vi "Periodic Tasks.vi"() -> ()   [LabVIEW 2011]
doc: "This VI runs in parallel to other tasks. It can contain as many user-defined periodic loops as you need. These can carry out PID or other sorts of timed response."
uses:
  <vilib>/Rock Robotics/SystemInterfaces/Utilities/FPGA_UtilitiesLED State.ctl
  <vilib>/Rock Robotics/SystemInterfaces/Utilities/FPGA_UtilitiesLED Source.ctl
  Robot Global Data.vi
  <vilib>/Rock Robotics/WPI/Relay/WPI_RelayValue.ctl
panel:
  in  "Speed of Harvester":dbl
  in  "Speed of Conveyor":dbl
  out "Rate 3":dbl
  out "error out 4":errorcluster
  out "Direction 3":bool
  out "Distance 3":dbl
  out "Distance 2":dbl
  out "Direction 2":bool
  out "error out 3":errorcluster
  out "Rate 2":dbl
  out "Rate":dbl
  out "error out 2":errorcluster
  out "I2C":bool
  out "Angular Rate":dbl
  out "Angle":dbl
  out "Direction":bool
  out "Distance":dbl
  # "Target Tracking"
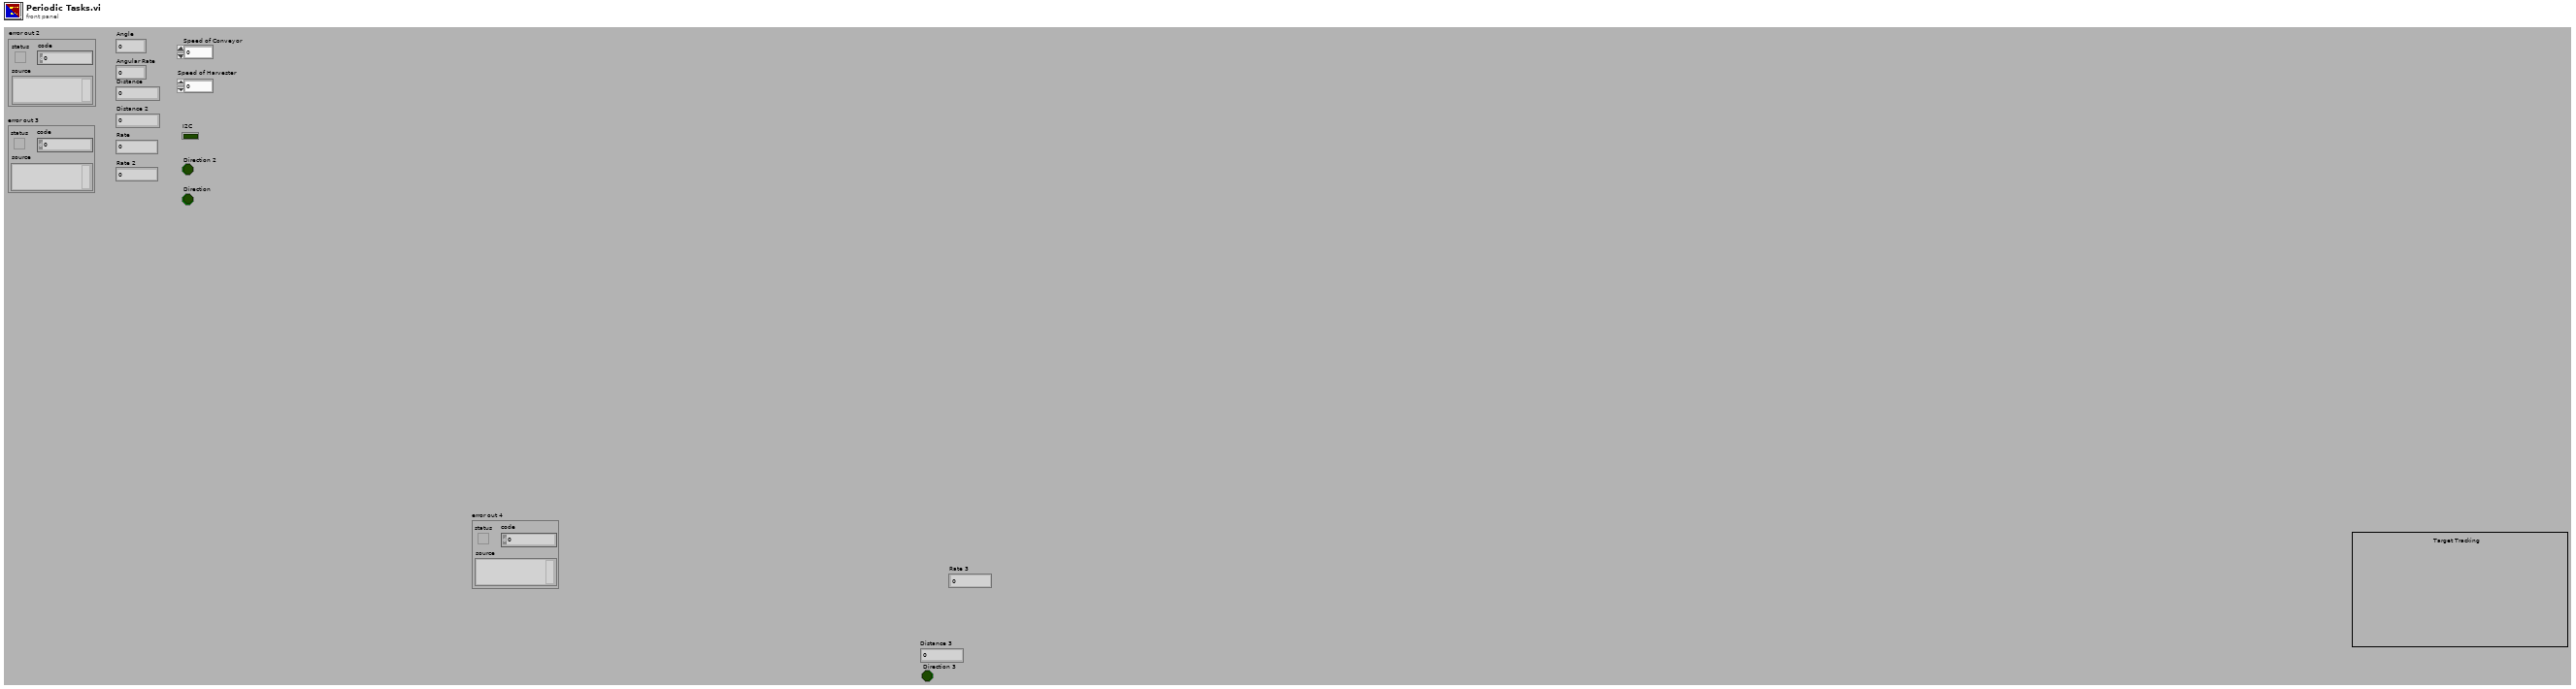
[diagram p1: front panel]
types:
  T1 = typedef "WPI_RelayValue.ctl" = enum16{"Off", "On", "Forward", "Reverse"}
  T2 = typedef "WPI_AnalogChannelDevRef.ctl" = cluster{"DevStatus":errorcluster, "Analog Module":T3, "Analog Channel":T4}
  T3 = typedef "FPGA_TypedefAnalogModule.ctl" = enum16{"Analog Module 1", "Analog Module 2"}
  T4 = typedef "FPGA_AIChannel.ctl" = enum8{"AI 1", "AI 2", "AI 3", "AI 4", "AI 5", "AI 6", "AI 7", "AI 8", "Invalid"}
  T5 = typedef "WPI_EncoderDevRef.ctl" = cluster{"DevStatus":errorcluster, "EncoderIndex":T6, "CounterIndex":T7, "DistancePerCount":dbl, "Decoding Type":T8}
  T6 = typedef "FPGA_EncoderIdx.ctl" = enum8{"Enc 0", "Enc 1", "Enc 2", "Enc 3", "Invalid"}
  T7 = typedef "FPGA_CounterCtrSystemIndex.ctl" = enum8{"Ctr 0", "Ctr 1", "Ctr 2", "Ctr 3", "Ctr 4", "Ctr 5", "Ctr 6", "Ctr 7", "Invalid"}
  T8 = typedef "WPI_EncoderType.ctl" = enum16{"1x", "2x", "4x"}
  T9 = typedef "WPI_RelayDevRef.ctl" = cluster{"DevStatus":errorcluster, "Relay Channel":T10, "Digital Module":T11, "Relay Direction":T12}
  T10 = typedef "FPGA_DIORelayChannel.ctl" = enum8{"Relay 1", "Relay 2", "Relay 3", "Relay 4", "Relay 5", "Relay 6", "Relay 7", "Relay 8", "Invalid"}
  T11 = typedef "FPGA_TypedefDigitalModule.ctl" = enum16{"Digital Module 1", "Digital Module 2"}
  T12 = typedef "WPI_RelayDirection.ctl" = enum16{"Both directions", "Forward only", "Reverse only"}
  T13 = typedef "WPI_GyroDevRef.ctl" = cluster{"DevStatus":errorcluster, "Analog Module":T3, "Analog Channel":T4, "Offset":dbl, "Gain (VoltsPerDegree/Second)":dbl}
  T14 = cluster{"Driver Station Digital Output (1-8)[0]":bool, "Driver Station Digital Output (1-8)[1]":bool, "Driver Station Digital Output (1-8)[2]":bool, "Driver Station Digital Output (1-8)[3]":bool, "Driver Station Digital Output (1-8)[4]":bool, "Driver Station Digital Output (1-8)[5]":bool, "Driver Station Digital Output (1-8)[6]":bool, "Driver Station Digital Output (1-8)[7]":bool, "Driver Station Digital Output (1-8)[8]":bool}
  T15 = typedef "FPGA_UtilitiesLED State.ctl" = enum16{"Off", "On", "Toggle"}
  T16 = typedef "FPGA_UtilitiesLED Source.ctl" = enum16{"User LED", "FPGA LED"}
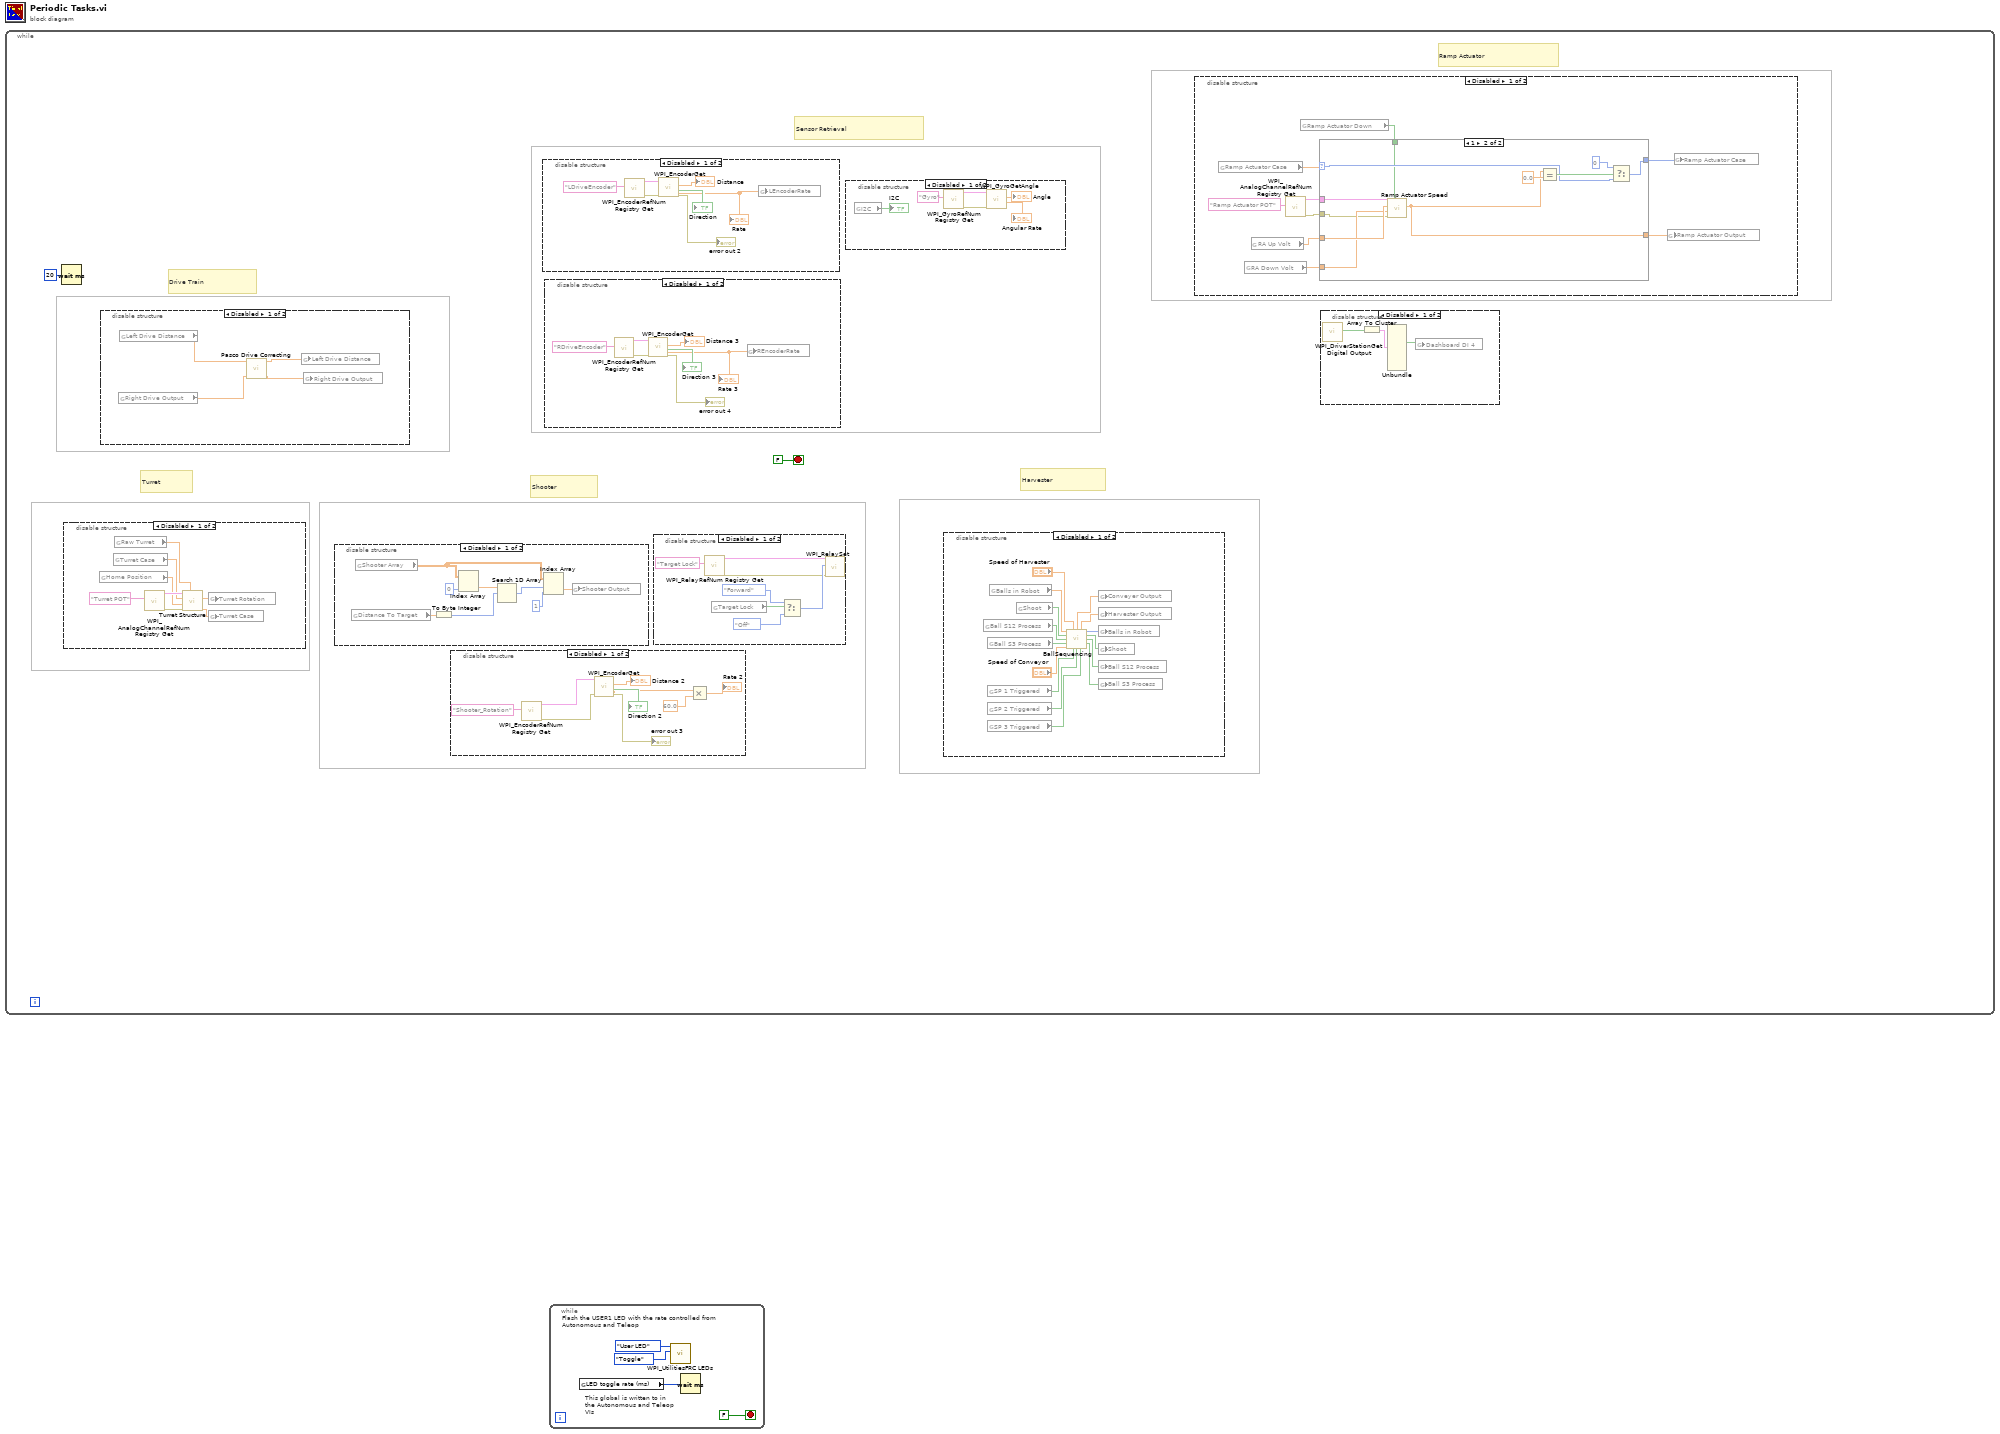
[diagram p0: block diagram]
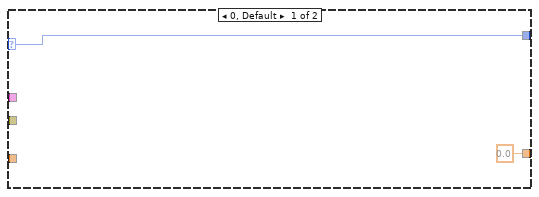
[diagram p4: hidden frame]
diagram:
  n1 = while {
    stop <- FALSE stop-if-true
    # "Harvester"
    # "Shooter"
    # "Sensor Retrieval"
    # "Turret"
    # "Drive Train"
    # "Ramp Actuator"
    n2 = Wait (ms)(milliseconds to wait=u32 20) -> ()  [unwired: 1 out]
    n3 = disable-structure shown="Disabled" {
      frame Disabled {
        n4 = global read "Robot Global Data.vi" "Home Position"() -> (w50:dbl)
        n5 = global read "Robot Global Data.vi" "Turret Case"() -> (w51:dbl)
        n6 = global read "Robot Global Data.vi" "Raw Turret"() -> (w49:dbl)
        n7 = call <vilib>:"WPI_AnalogChannelRefNum Registry Get.vi"("refnum name"="Turret POT") -> ("error out"=w52:errorcluster, "AIDeviceRef"=w53:T2)  [unwired: 9 in]
        n8 = call "Turret Structure.vi"("Raw Turret"=w49, "error in (no error)"=w52, "Home postion"=w50, "Turret Case"=w51, "AIDeviceRef"=w53) -> ("Turret Case Output"=w47:dbl, "Turret Output"=w48:dbl)  [unwired: 5 in]
        n9 = global write "Robot Global Data.vi" "Turret Rotation"(w48) -> ()
        n10 = global write "Robot Global Data.vi" "Turret Case"(w47) -> ()
      }
      frame Enabled {
      }
    }
    n11 = disable-structure shown="Disabled" {
      frame Disabled {
        n12 = global read "Robot Global Data.vi" "Right Drive Output"() -> (w65:dbl)
        n13 = global read "Robot Global Data.vi" "Left Drive Distance"() -> (w66:dbl)
        n14 = call "Pasco Drive Correcting.vi"("RightDriveOutput"=w65, "LeftDriveOutput"=w66) -> ("RightDriveOutput"=w63:dbl, "LeftDriveOutput"=w64:dbl)  [unwired: 8 in]
        n15 = global write "Robot Global Data.vi" "Left Drive Distance"(w64) -> ()
        n16 = global write "Robot Global Data.vi" "Right Drive Output"(w63) -> ()
      }
      frame Enabled {
      }
    }
    n17 = disable-structure shown="Disabled" {
      frame Disabled {
        n18 = global read "Robot Global Data.vi" "Distance To Target"() -> (w60:dbl)
        n19 = global read "Robot Global Data.vi" "Shooter Array"() -> (w58:dbl[][])
        n20 = To Byte Integer(number=w60) -> (8bit integer=w59:i8)
        n21 = Index Array(array=w58, index (col)=0 ("disabled index (col)")) -> (element=w61:dbl[])  [unwired: 1 in]
        n22 = Search 1D Array(1D array=w61, element=w59) -> (index of element=w57:i32)  [unwired: 1 in]
        n23 = Index Array(array=w58, index (row)=w57, index (col)=1 ("disabled index (col)")) -> (element=w55:dbl)
        n24 = global write "Robot Global Data.vi" "Shooter Output"(w55) -> ()
      }
      frame Enabled {
      }
    }
    n25 = disable-structure shown="Disabled" {
      frame Disabled {
        n26 = call <vilib>:"WPI_EncoderRefNum Registry Get.vi"("refnum name"="Shooter_Rotation") -> ("error out"=w90:errorcluster, "EncoderDevRef"=w91:T5)  [unwired: 9 in]
        n27 = call <vilib>:"WPI_EncoderGet.vi"("error in (no error)"=w90, "EncoderDevRef"=w91) -> ("error out"=→"error out 3":errorcluster, "Direction"=→"Direction 2":bool, "Distance"=→"Distance 2":dbl, "Rate"=w94:dbl)  [unwired: 4 in, 2 out]
        n28 = Multiply(x=w94, y=60.0) -> (x*y=→"Rate 2":dbl)
      }
      frame Enabled {
      }
    }
    n29 = disable-structure shown="Disabled" {
      frame Disabled {
        n30 = call <vilib>:"WPI_EncoderRefNum Registry Get.vi"("refnum name"="LDriveEncoder") -> ("error out"=w81:errorcluster, "EncoderDevRef"=w80:T5)  [unwired: 9 in]
        n31 = call <vilib>:"WPI_EncoderGet.vi"("error in (no error)"=w81, "EncoderDevRef"=w80) -> ("error out"=→"error out 2":errorcluster, "Direction"=→"Direction":bool, "Distance"=→"Distance":dbl, "Rate"=w77:dbl)  [unwired: 4 in, 2 out]
        "Rate" <- w77
        n32 = global write "Robot Global Data.vi" "LEncoderRate"(w77) -> ()
      }
      frame Enabled {
      }
    }
    n33 = disable-structure shown="Disabled" {
      frame Disabled {
        n34 = call <vilib>:"WPI_EncoderRefNum Registry Get.vi"("refnum name"="RDriveEncoder") -> ("error out"=w74:errorcluster, "EncoderDevRef"=w73:T5)  [unwired: 9 in]
        n35 = call <vilib>:"WPI_EncoderGet.vi"("error in (no error)"=w74, "EncoderDevRef"=w73) -> ("error out"=→"error out 4":errorcluster, "Direction"=→"Direction 3":bool, "Distance"=→"Distance 3":dbl, "Rate"=w70:dbl)  [unwired: 4 in, 2 out]
        "Rate 3" <- w70
        n36 = global write "Robot Global Data.vi" "REncoderRate"(w70) -> ()
      }
      frame Enabled {
      }
    }
    n37 = disable-structure shown="Disabled" {
      frame Disabled {
        n38 = call <vilib>:"WPI_RelayRefNum Registry Get.vi"("refnum name"="Target Lock") -> ("error out"=w18:errorcluster, "RelayDevRef"=w19:T9)  [unwired: 9 in]
        n39 = global read "Robot Global Data.vi" "Target Lock"() -> (w24:bool)
        n40 = Select(t=WPI_RelayValue."Forward" ("RelayValue"), s=w24, f=WPI_RelayValue."Off" ("RelayValue")) -> (s? t:f=w21:T1)
        n41 = call <vilib>:"WPI_RelaySet.vi"("error in (no error)"=w18, "RelayValue"=w21, "RelayDevRef"=w19) -> ()  [unwired: 7 in, 2 out]
      }
      frame Enabled {
      }
    }
    n42 = disable-structure shown="Disabled" {
      frame Disabled {
        n43 = global read "Robot Global Data.vi" "I2C"() -> (→"I2C":bool)
        n44 = call <vilib>:"WPI_GyroRefNum Registry Get.vi"("refnum name"="Gyro") -> ("error out"=w88:errorcluster, "GyroDevRef"=w89:T13)  [unwired: 9 in]
        n45 = call <vilib>:"WPI_GyroGetAngle.vi"("error in (no error)"=w88, "GyroDevRef"=w89) -> ("Angular Rate"=→"Angular Rate":dbl, "Angle"=→"Angle":dbl)  [unwired: 6 in, 2 out]
      }
      frame Enabled {
      }
    }
    n46 = disable-structure shown="Disabled" {
      frame Disabled {
        n47 = global read "Robot Global Data.vi" "Ball S12 Process"() -> (w4:bool)
        n48 = global read "Robot Global Data.vi" "Ball S3 Process"() -> (w3:bool)
        n49 = global read "Robot Global Data.vi" "SP 1 Triggered"() -> (w11:bool)
        n50 = global read "Robot Global Data.vi" "SP 2 Triggered"() -> (w12:bool)
        n51 = global read "Robot Global Data.vi" "SP 3 Triggered"() -> (w13:bool)
        n52 = global read "Robot Global Data.vi" "Balls in Robot"() -> (w6:dbl)
        n53 = global read "Robot Global Data.vi" "Shoot"() -> (w5:bool)
        n54 = call "BallSequencing.vi"("Balls In Robot"=w6, "Speed of Harvester"="Speed of Harvester", "Shoot"=w5, "Ball S12 Process"=w4, "Ball S3 Process"=w3, "Speed of Conveyor"="Speed of Conveyor", "SP 1 Triggered"=w11, "SP 2 Triggered"=w12, "SP 3 Triggered"=w13) -> ("Conveyer Output"=w7:dbl, "Harvester Output"=w8:dbl, "Balls In Robot Output"=w17:i32, "Shoot Output"=w16:bool, "Ball S12 Process Output"=w15:bool, "Ball S3 Process Output"=w14:bool)  [unwired: 1 in]
        n55 = global write "Robot Global Data.vi" "Conveyer Output"(w7) -> ()
        n56 = global write "Robot Global Data.vi" "Harvester Output"(w8) -> ()
        n57 = global write "Robot Global Data.vi" "Balls in Robot"(w17) -> ()
        n58 = global write "Robot Global Data.vi" "Shoot"(w16) -> ()
        n59 = global write "Robot Global Data.vi" "Ball S12 Process"(w15) -> ()
        n60 = global write "Robot Global Data.vi" "Ball S3 Process"(w14) -> ()
      }
      frame Enabled {
      }
    }
    n61 = disable-structure shown="Disabled" {
      frame Disabled {
        n62 = global read "Robot Global Data.vi" "Ramp Actuator Case"() -> (w33:dbl)
        n63 = global read "Robot Global Data.vi" "RA Down Volt"() -> (w28:dbl)
        n64 = global read "Robot Global Data.vi" "RA Up Volt"() -> (w29:dbl)
        n65 = call <vilib>:"WPI_AnalogChannelRefNum Registry Get.vi"("refnum name"="Ramp Actuator POT") -> ("error out"=w26:errorcluster, "AIDeviceRef"=w27:T2)  [unwired: 9 in]
        n66 = global read "Robot Global Data.vi" "Ramp Actuator Down"() -> (w25:bool)
        n67 = case shown="1" w33 {
          selector: w33 -> [w35 w40]
          tunnel: [w35 w37] -> w32
          tunnel: [0.0 ("f") w38] -> w30
          tunnel: w29 -> [_ w46]
          tunnel: w28 -> [_ w45]
          tunnel: w27 -> [_ w44]
          tunnel: w26 -> [_ w43]
          tunnel: w25 -> [_ w36]
          frame 0, Default {
          }
          frame 1 {
            n68 = call "Ramp Actuator Speed.vi"("Up to Down"=w36, "error in (no error)"=w43, "RA Down Volt"=w45, "RA Up Volt"=w46, "AIDeviceRef"=w44) -> ("Ramp Actuator Ouput"=w38:dbl)  [unwired: 6 in]
            n69 = Equal?(x=w38, y=0.0) -> (x = y?=w41:bool)
            n70 = Select(t=0, s=w41, f=w40) -> (s? t:f=w37:i32)
          }
        }
        n71 = global write "Robot Global Data.vi" "Ramp Actuator Output"(w30) -> ()
        n72 = global write "Robot Global Data.vi" "Ramp Actuator Case"(w32) -> ()
      }
      frame Enabled {
      }
    }
    n73 = disable-structure shown="Disabled" {
      frame Disabled {
        n74 = call <vilib>:"WPI_DriverStationGet Digital Output.vi"() -> ("Driver Station Digital Output (1-8)"=w69:bool[])  [unwired: 10 in, 1 out]
        n75 = Array To Cluster(array=w69) -> (cluster=w68:T14)
        n76 = Unbundle(w68) -> ("Driver Station Digital Output (1-8)[3]"=w67:bool)  [unwired: 8 out]
        n77 = global write "Robot Global Data.vi" "Dashboard DI 4"(w67) -> ()
      }
      frame Enabled {
      }
    }
  }
  n78 = while {
    stop <- FALSE stop-if-true
    # "This global is written to in the Autonomous and Teleop VIs"
    # "Flash the USER1 LED with the rate controlled from Autonomous and Teleop"
    n79 = global read "Robot Global Data.vi" "LED toggle rate (ms)"() -> (w99:u32)
    n80 = call <vilib>:"WPI_UtilitiesFRC LEDs.vi"("State"=FPGA_UtilitiesLED_State."Toggle", "LED Type"=FPGA_UtilitiesLED_Source."User LED") -> ()  [unwired: 1 in, 9 out]
    n81 = Wait (ms)(milliseconds to wait=w99) -> ()  [unwired: 1 out]
  }
